vi "Command Panel.vi"(8 "error in (no error)":errorcluster, 10 "command":string, 11 "VISA resource name":refnum<visa-resource-name>="COM4") -> (0 "error out":errorcluster)   [LabVIEW 2017]
uses:
  <vilib>/Instr/_visa.llb/VISA Flush IO Buffer Mask.ctl
  <vilib>/Instr/_visa.llb/VISA Configure Serial Port (Instr).vi
panel:
  out "read buffer":string
  out "read buffer 2":string
  in  "Query":string="W"
  in  "Query":bool
  in  "Set":bool
  in  "Clear":bool
  out "error mid (no error) 2":errorcluster
  in  "stop":bool
  in  "Write":bool
  in  "Read":bool
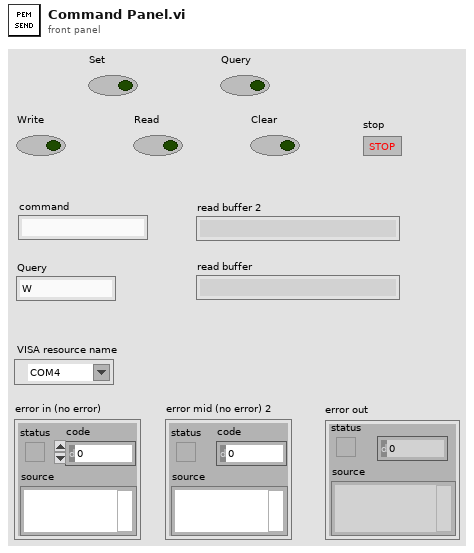
[diagram p1: front panel]
types:
  T1 = typedef "VISA Flush IO Buffer Mask.ctl" = u16
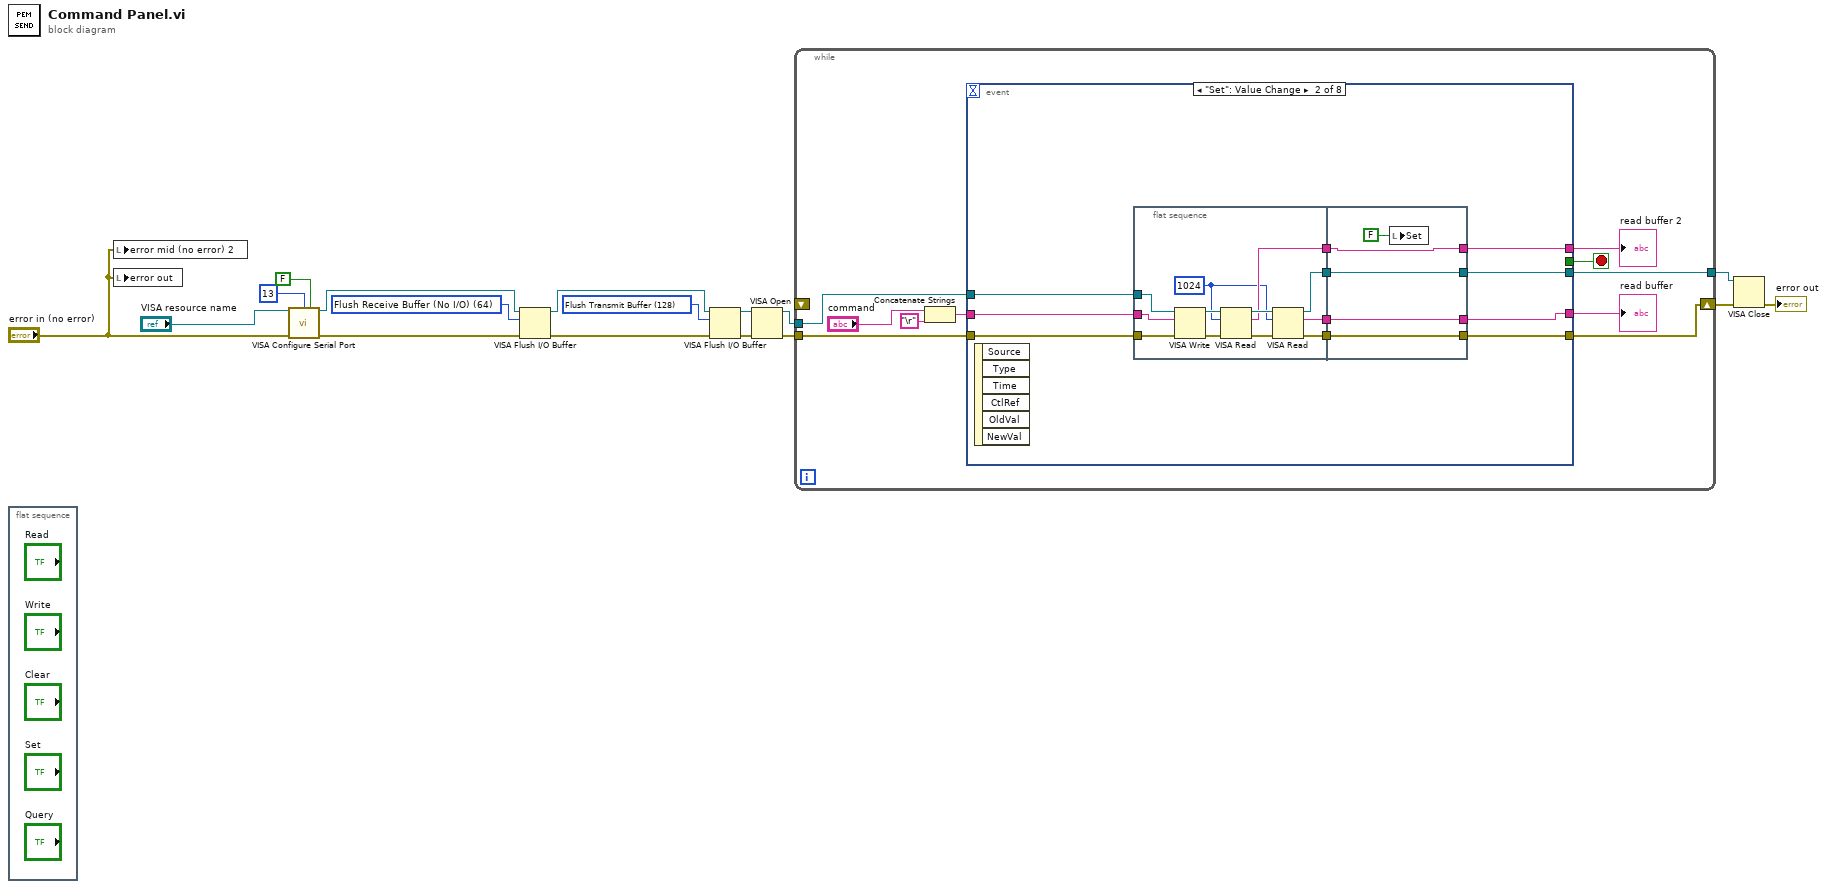
[diagram p0: block diagram]
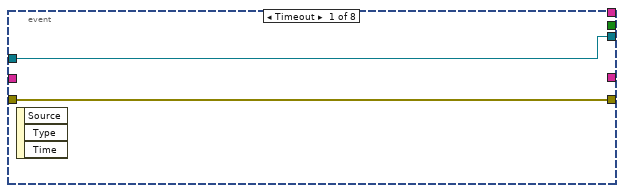
[diagram p2: hidden frame]
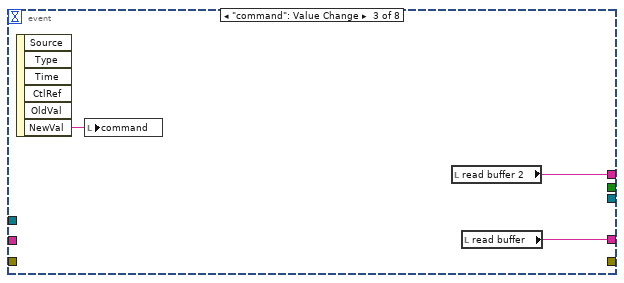
[diagram p3: hidden frame]
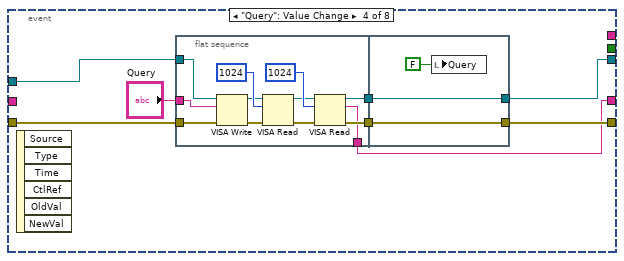
[diagram p4: hidden frame]
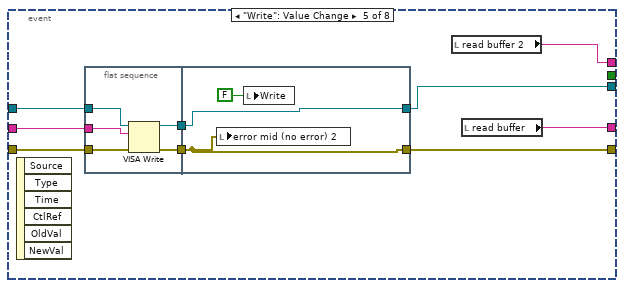
[diagram p5: hidden frame]
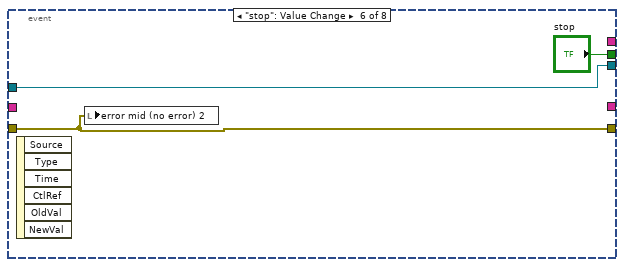
[diagram p6: hidden frame]
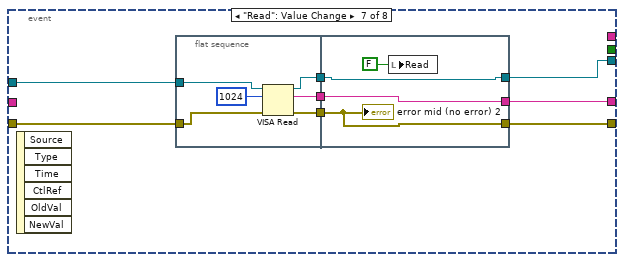
[diagram p7: hidden frame]
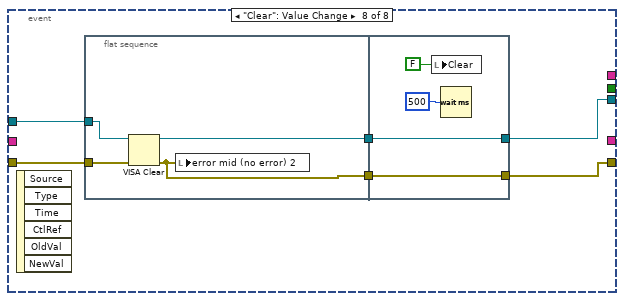
[diagram p8: hidden frame]
diagram:
  w7 = T1 64 items=["Flush Receive Buffer"=16, "Write Transmit Buffer to Device"=32, "Flush Receive Buffer (No I/O)"=64, "Flush Transmit Buffer"=128] ("Mask")
  w8 = T1 128 items=["Flush Receive Buffer"=16, "Write Transmit Buffer to Device"=32, "Flush Receive Buffer (No I/O)"=64, "Flush Transmit Buffer"=128] ("Mask")
  n1 = flat-sequence {
    frame #0 {
    }
  }
  n2 = local write "error mid (no error) 2"("error in (no error)") -> ()
  n3 = local write "error out"("error in (no error)") -> ()
  n4 = call-poly "VISA Configure Serial Port"("VISA resource name"="VISA resource name", "termination char\n(0xA = '\\n' = LF)"=u8 13 ("termination char\n(0xA = '\\n' = LF)"), "Enable Termination\nChar (T)"=FALSE ("Enable Termination\nChar (T)"), "error in (no error)"="error in (no error)") -> ("VISA resource name out"=w10:refnum<visa-resource-name>, "error out"=w11:errorcluster)  [unwired: 10 in]
  n5 = VISA Flush I/O Buffer(VISA resource name=w10, mask (16)=w7, error in (no error)=w11) -> (VISA resource name out=w9:refnum<visa-resource-name>, error out=w12:errorcluster)
  n6 = VISA Flush I/O Buffer(VISA resource name=w9, mask (16)=w8, error in (no error)=w12) -> (VISA resource name out=w5:refnum<visa-resource-name>, error out=w4:errorcluster)
  n7 = VISA Open(error in (no error)=w4, VISA resource name=w5) -> (VISA resource name=w13:refnum<visa-resource-name>, error out=w14:errorcluster)  [unwired: 3 in]
  n8 = while {
    tunnel: [w25] -> w17
    shift-right: [w26] -> w16
    shift-left: _ -> [_]
    tunnel: w14 -> [w22]
    tunnel: w13 -> [w21]
    stop <- w27 stop-if-true
    n9 = Concatenate Strings("command", "\r") -> (w23:string)
    n10 = event shown="[1] \"Set\": Value Change" {
      selector: _ -> [_ _ _ _ _ _ _ _]
      dyn-events: _ -> [_ _ _ _ _ _ _ _]
      timeout: _ -> [_ _ _ _ _ _ _ _]
      tunnel: [_ _ _ _ _ "stop" _ _] -> w27
      tunnel: w22 -> [w29 w37 _ w64 w92 w101 w111 w126]
      tunnel: w23 -> [_ w36 _ _ w91 _ _ _]
      tunnel: w21 -> [w28 w38 _ w65 w90 w102 w108 w127]
      tunnel: [w29 w39 _ w62 w89 w101 w110 w124] -> w26
      tunnel: [w28 w40 _ w63 w88 w102 w107 w125] -> w25
      tunnel: [_ w32 w60 w61 w85 _ w109 _] -> w19
      tunnel: [_ w31 w58 _ w84 _ _ _] -> w20
      event Timeout {
        n11 = event-data() -> ()  [unwired: 1 in, 3 out]
      }
      event "Set": Value Change {
        n12 = event-data() -> ()  [unwired: 1 in, 6 out]
        n13 = flat-sequence {
          tunnel: w38 -> [w48]
          tunnel: w37 -> [w47]
          tunnel: w36 -> [w46]
          tunnel: [w42] -> w35
          tunnel: [w43] -> w34
          tunnel: [w45] -> w33
          tunnel: [w44] -> w30
          tunnel: [w56] -> w39
          tunnel: [w57] -> w40
          tunnel: w35 -> [w57]
          tunnel: w34 -> [w56]
          tunnel: [w54] -> w32
          tunnel: w33 -> [w54]
          tunnel: [w53] -> w31
          tunnel: w30 -> [w53]
          frame #0 {
            w41 = u32 1024 ("byte count")
            n14 = VISA Write(VISA resource name=w48, write buffer=w46, error in (no error)=w47) -> (VISA resource name out=w52:refnum<visa-resource-name>, error out=w51:errorcluster)  [unwired: 1 out]
            n15 = VISA Read(VISA resource name=w52, byte count=w41, error in (no error)=w51) -> (VISA resource name out=w49:refnum<visa-resource-name>, read buffer=w44:string, error out=w50:errorcluster)  [unwired: 1 out]
            n16 = VISA Read(VISA resource name=w49, byte count=w41, error in (no error)=w50) -> (VISA resource name out=w42:refnum<visa-resource-name>, read buffer=w45:string, error out=w43:errorcluster)  [unwired: 1 out]
          }
          frame #1 {
            n17 = local write "Set"(FALSE ("Set")) -> ()
          }
        }
      }
      event "command": Value Change {
        n18 = event-data() -> ("NewVal"=w59:string)  [unwired: 1 in, 5 out]
        n19 = local write "command"(w59) -> ()
        n20 = local read "read buffer 2"() -> (w58:string)
        n21 = local read "read buffer"() -> (w60:string)
      }
      event "Query": Value Change {
        n22 = event-data() -> ()  [unwired: 1 in, 6 out]
        n23 = flat-sequence {
          tunnel: w65 -> [w72]
          tunnel: w64 -> [w71]
          tunnel: "Query" -> [w70]
          tunnel: [w74] -> w68
          tunnel: [w73] -> w67
          tunnel: [w69] -> w61
          tunnel: [w82] -> w62
          tunnel: [w83] -> w63
          tunnel: w68 -> [w83]
          tunnel: w67 -> [w82]
          frame #0 {
            n24 = VISA Write(VISA resource name=w72, write buffer=w70, error in (no error)=w71) -> (VISA resource name out=w78:refnum<visa-resource-name>, error out=w77:errorcluster)  [unwired: 1 out]
            n25 = VISA Read(VISA resource name=w78, byte count=u32 1024, error in (no error)=w77) -> (VISA resource name out=w75:refnum<visa-resource-name>, error out=w76:errorcluster)  [unwired: 2 out]
            n26 = VISA Read(VISA resource name=w75, byte count=u32 1024, error in (no error)=w76) -> (VISA resource name out=w74:refnum<visa-resource-name>, read buffer=w69:string, error out=w73:errorcluster)  [unwired: 1 out]
          }
          frame #1 {
            n27 = local write "Query"(FALSE ("Query")) -> ()
          }
        }
      }
      event "Write": Value Change {
        n28 = event-data() -> ()  [unwired: 1 in, 6 out]
        n29 = flat-sequence {
          tunnel: w92 -> [w97]
          tunnel: w91 -> [w96]
          tunnel: w90 -> [w95]
          tunnel: [w94] -> w87
          tunnel: [w93] -> w86
          tunnel: [w100] -> w88
          tunnel: [w98] -> w89
          tunnel: w87 -> [w98]
          tunnel: w86 -> [w100]
          frame #0 {
            n30 = VISA Write(VISA resource name=w95, write buffer=w96, error in (no error)=w97) -> (VISA resource name out=w93:refnum<visa-resource-name>, error out=w94:errorcluster)  [unwired: 1 out]
          }
          frame #1 {
            n31 = local write "error mid (no error) 2"(w98) -> ()
            n32 = local write "Write"(FALSE ("Write")) -> ()
          }
        }
        n33 = local read "read buffer 2"() -> (w84:string)
        n34 = local read "read buffer"() -> (w85:string)
      }
      event "stop": Value Change {
        n35 = event-data() -> ()  [unwired: 1 in, 6 out]
        n36 = local write "error mid (no error) 2"(w101) -> ()
      }
      event "Read": Value Change {
        n37 = event-data() -> ()  [unwired: 1 in, 6 out]
        n38 = flat-sequence {
          tunnel: w111 -> [w116]
          tunnel: w108 -> [w113]
          tunnel: [w115] -> w106
          tunnel: [w114] -> w105
          tunnel: [w112] -> w104
          tunnel: [w120] -> w107
          tunnel: [w121] -> w109
          tunnel: [w118] -> w110
          tunnel: w106 -> [w118]
          tunnel: w105 -> [w121]
          tunnel: w104 -> [w120]
          frame #0 {
            n39 = VISA Read(VISA resource name=w113, byte count=u32 1024, error in (no error)=w116) -> (VISA resource name out=w112:refnum<visa-resource-name>, read buffer=w114:string, error out=w115:errorcluster)  [unwired: 1 out]
          }
          frame #1 {
            n40 = local write "Read"(FALSE ("Read")) -> ()
            "error mid (no error) 2" <- w118
          }
        }
      }
      event "Clear": Value Change {
        n41 = event-data() -> ()  [unwired: 1 in, 6 out]
        n42 = flat-sequence {
          tunnel: w127 -> [w131]
          tunnel: w126 -> [w130]
          tunnel: [w129] -> w123
          tunnel: [w128] -> w122
          tunnel: [w134] -> w124
          tunnel: [w135] -> w125
          tunnel: w123 -> [w135]
          tunnel: w122 -> [w134]
          frame #0 {
            n43 = VISA Clear(VISA resource name=w131, error in (no error)=w130) -> (VISA resource name out=w129:refnum<visa-resource-name>, error out=w128:errorcluster)
            n44 = local write "error mid (no error) 2"(w128) -> ()
          }
          frame #1 {
            n45 = local write "Clear"(FALSE ("Clear")) -> ()
            n46 = Wait (ms)(milliseconds to wait=u32 500) -> ()  [unwired: 1 out]
          }
        }
      }
    }
    "read buffer 2" <- w20
    "read buffer" <- w19
  }
  n47 = VISA Close(VISA resource name=w17, error in (no error)=w16) -> (error out=→"error out":errorcluster)
